vi "SubPanel_DataCollection_Rev11_v6.vi"(0 "DCPowerInformationClusterArray_Input":T6(array[cluster]), 1 "VISAPowerInfoInputArray":T5(array[cluster]), 2 "Run Data SubPanel Input":T4, 3 "RF Block Parameters":T3, 4 "Oscilloscope Info Array":T2(array[cluster]) {"vertical coupling" items=["AC", "DC", "Ground"]}, 6 "New Run?":bool, 7 "error in":errorcluster) -> (20 "DCPowerInformationClusterArray_Output":T6(array[cluster]), 21 "VISAPowerInfoInputOutput":T5(array[cluster]), 22 "Run Data SubPanel Output":T4, 23 "RF Block Parameters Output":T3, 24 "Oscilloscope Info Array Output":T2(array[cluster]) {"vertical coupling" items=["AC", "DC", "Ground"]}, 25 "Reinitialize?":bool, 26 "Data Was Collected?":bool, 27 "error out":errorcluster)   [LabVIEW 2019]
uses:
  Controls/DataBlockControl.ctl
  Controls/QueueDataControl_V3.ctl
  <vilib>/Utility/file.llb/Write Delimited Spreadsheet (string).vi
  Controls/RFBlockControl.ctl
  <instrlib>/niScope/Controls/niScope vertical coupling.ctl
panel:
  out "DCPowerInfoArray":string[][](array[string])
  out "Array":string[][][](array[string])
  out "Current Measurements":cluster{dbl[], dbl[]}[](graph)
  out "Voltage Measurements":cluster{dbl[], dbl[]}[](graph)
  out "Exiting":bool
  out "Full Run Information":string
  out "Ready For Next Run?":bool
  in  "Next Run":bool
  out "Recording Data":bool
  out "Current 2":waveform(dbl)[](graph)
  out "Voltage 2":waveform(dbl)[](graph)
  in  "Record Data Toggle":bool
  out "error of collection":errorcluster
  in  "force exit SubVI":bool
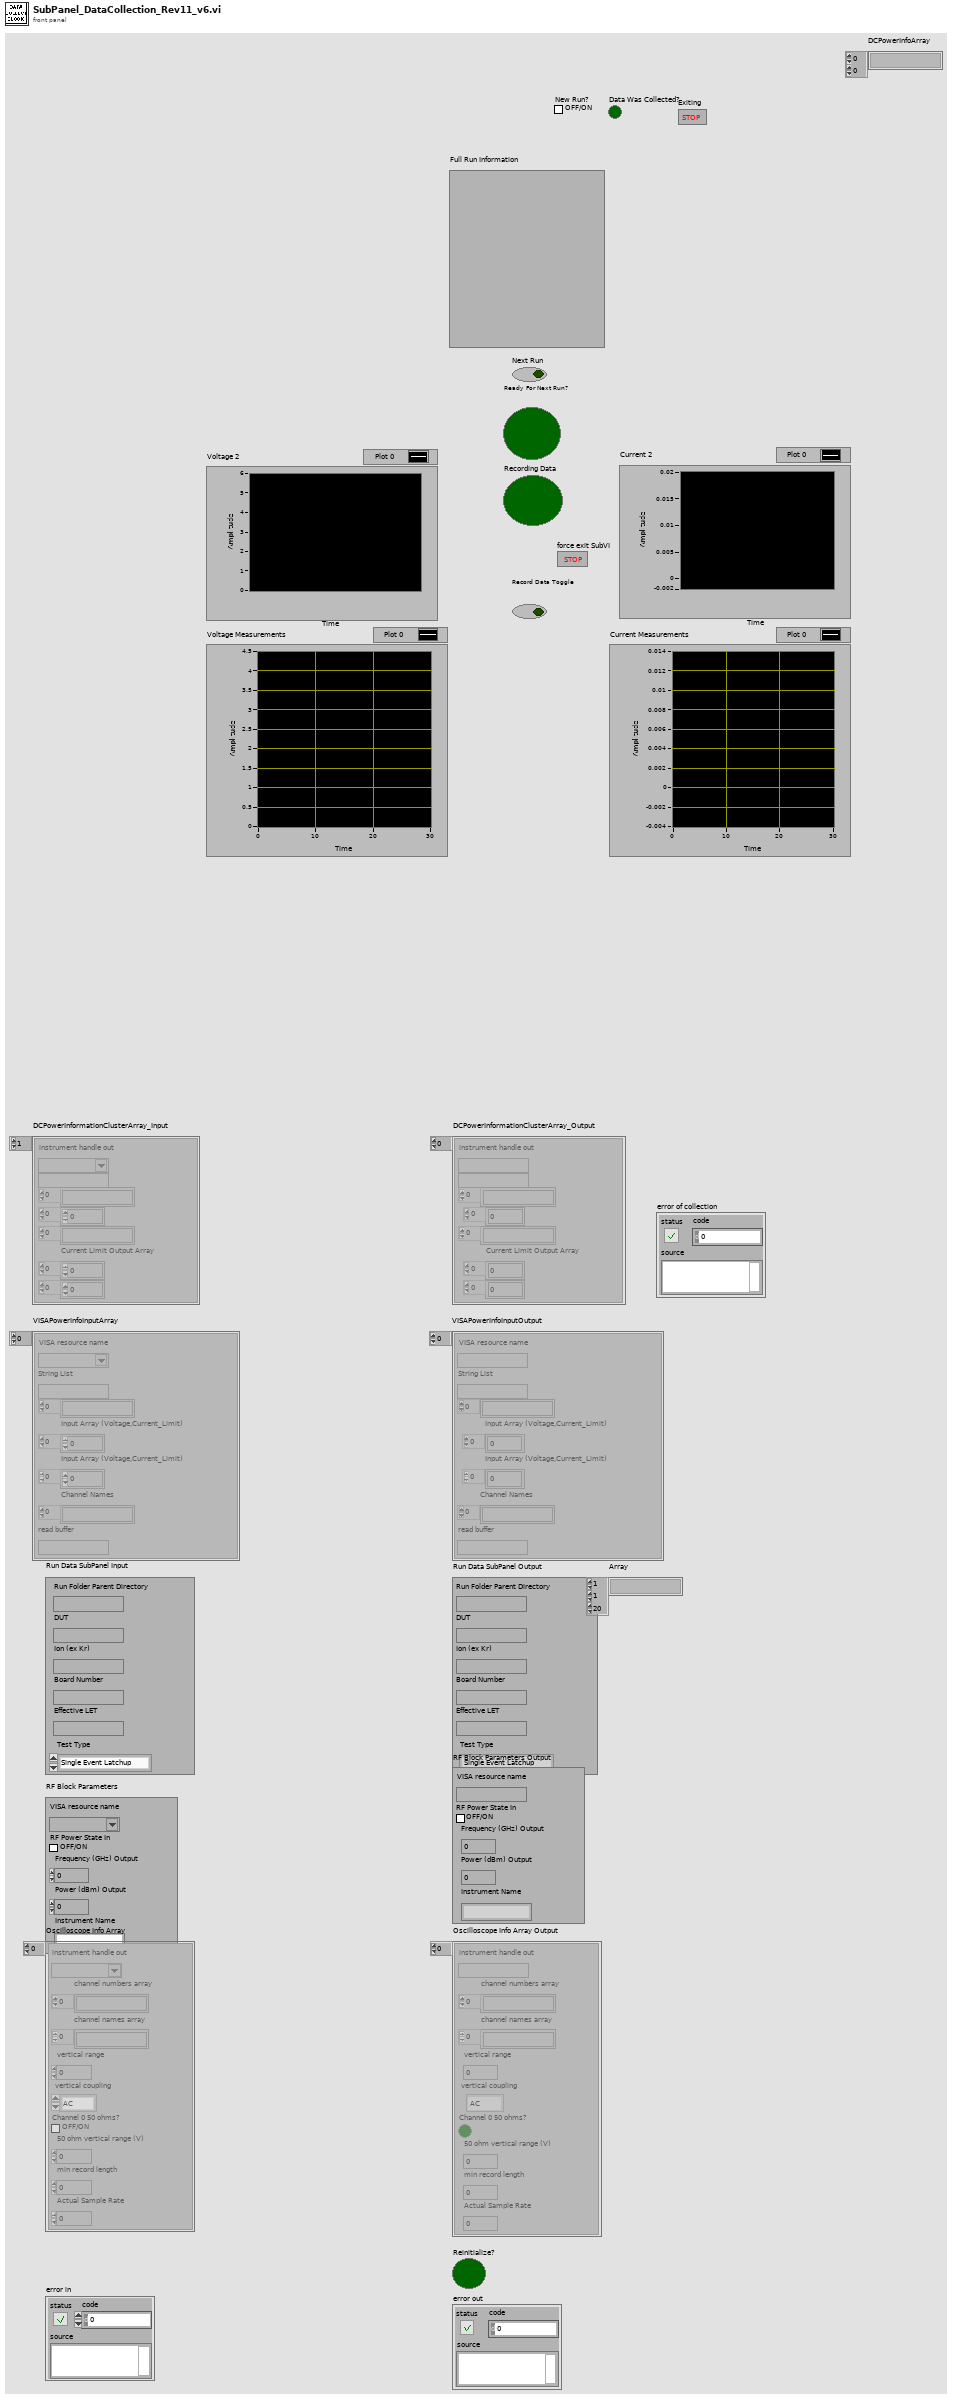
[diagram p1: front panel]
types:
  T1 = typedef "niScope vertical coupling.ctl" = i32
  T2 = cluster{"instrument handle out":refnum<k15>, "channel numbers array":string[], "channel names array":string[], "vertical range":dbl, "vertical coupling":T1, "Channel 0 50 ohms?":bool, "50 ohm vertical range (V)":dbl, "min record length":i32, "Actual Sample Rate":dbl}[]
  T3 = typedef "RFBlockControl.ctl" = cluster{"VISA resource name":refnum<visa-resource-name>, "RF Power State In":bool, "Frequency (GHz) Output":dbl, "Power (dBm) Output":dbl, "Instrument Name":string}
  T4 = typedef "DataBlockControl.ctl" = cluster{"Run Folder Parent Directory":path, "DUT":string, "Ion (ex Kr)":string, "Board Number":string, "Effective LET":string, "Test Type":enum16{"Single Event Latchup", "Single Event Transient", "Single Event Upset"}}
  T5 = cluster{"VISA resource name":refnum<visa-resource-name>, "String List":string, string[], "Input Array (Voltage,Current_Limit)":dbl[], "Input Array (Voltage,Current_Limit)":dbl[], "Channel Names":string[], "read buffer":string}[]
  T6 = cluster{"instrument handle out":refnum<k15>, string, string[], dbl[], string[], "Current Limit Output Array":dbl[], dbl[]}[]
  T7 = typedef "QueueDataControl_V3.ctl" = cluster{"Array of fetched data":dbl[][][], "Channel Names Array":string[], "Voltage Waveform Array":waveform(dbl)[], "Current Waveform Array":waveform(dbl)[], "Resetting Time":timestamp, "Beam Logic":dbl}
  T8 = cluster{"IVI Refnum out":refnum<k15>, string, "voltage level channel 23":dbl, "Channel Name 23":string, "Current Limit":dbl, "Measure Record dt":dbl, string}[]
  T9 = cluster{"created path":path, "DCPowerInformation_byChannel":cluster{"IVI Refnum out":refnum<k15>, string, "voltage level channel 23":dbl, "Channel Name 23":string, "Current Limit":dbl, "Measure Record dt":dbl, string}[], string[]}
  T10 = cluster{"Array of fetched data":dbl[][], string, i32[]}
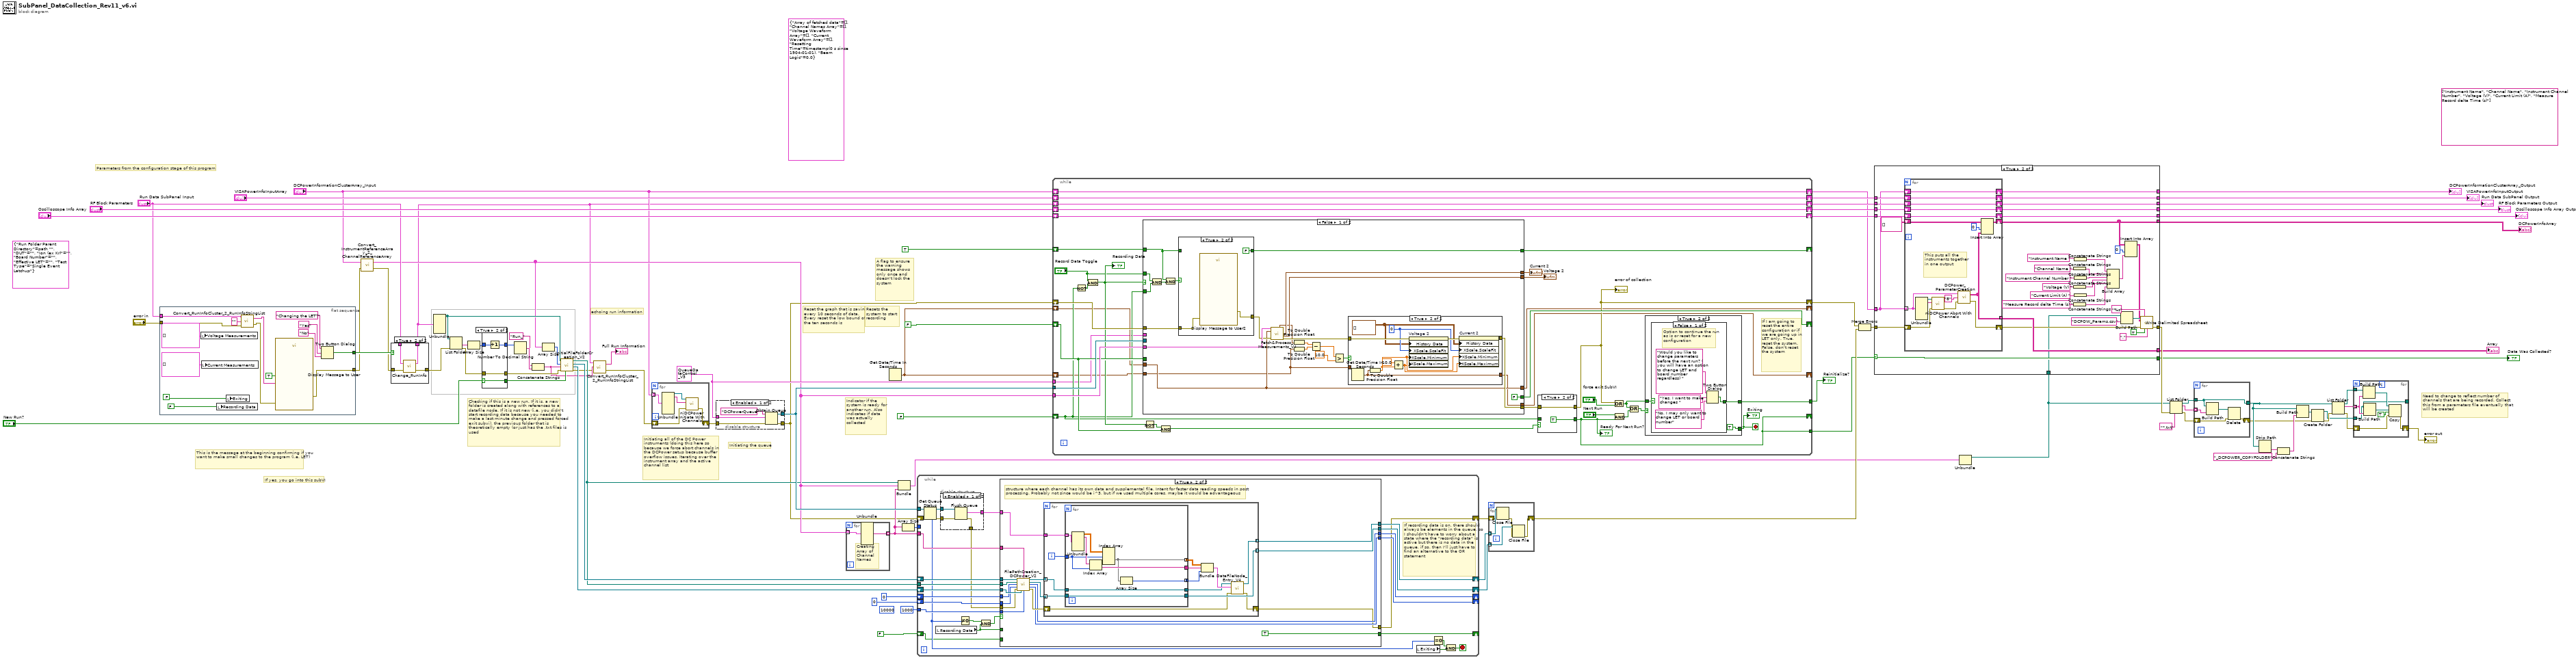
[diagram p0: block diagram]
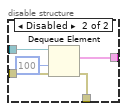
[diagram p2: hidden frame]
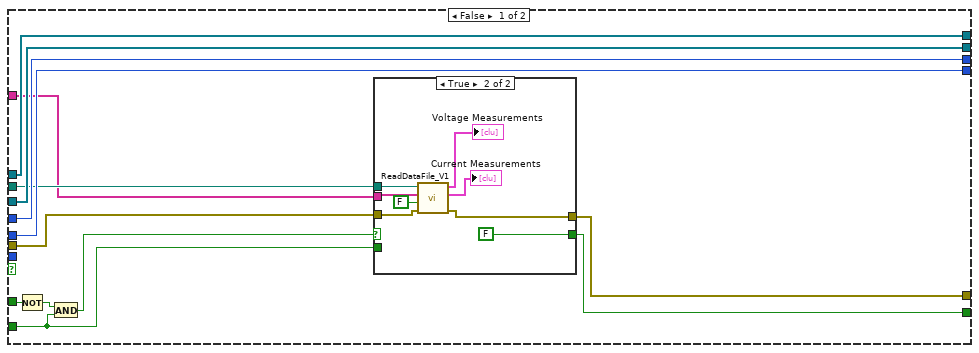
[diagram p3: hidden frame]
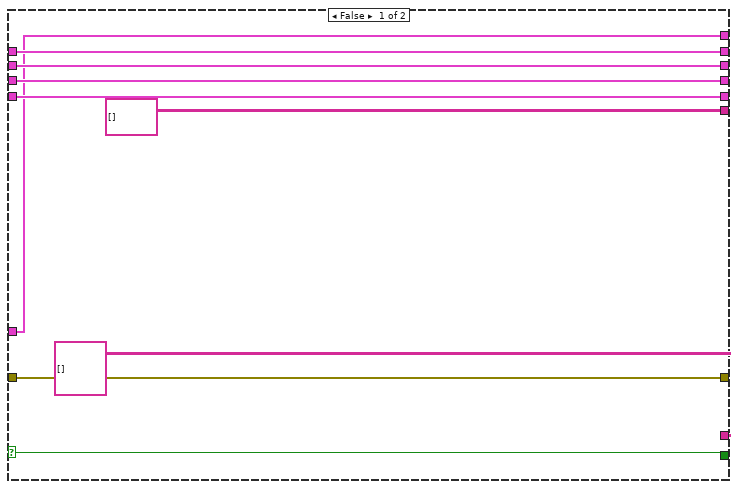
[diagram p5: hidden frame]
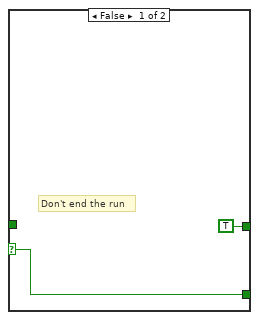
[diagram p9: hidden frame]
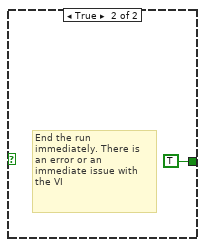
[diagram p10: hidden frame]
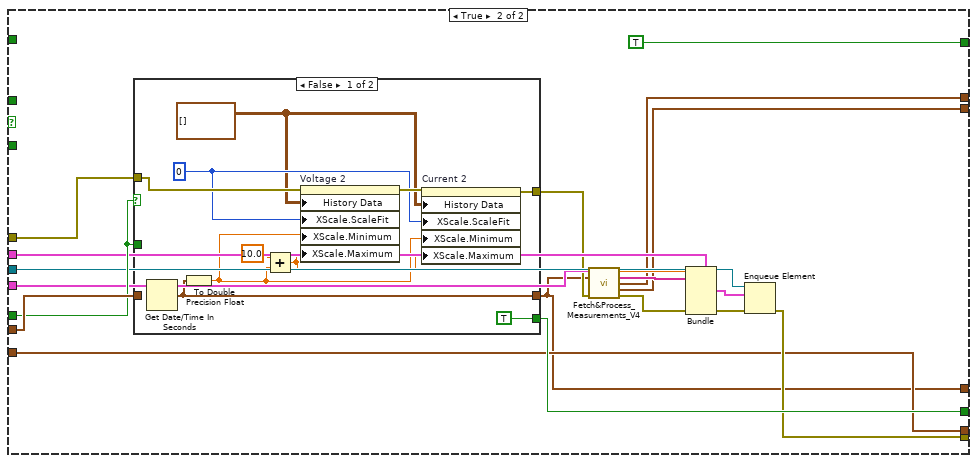
[diagram p14: hidden frame]
diagram:
  (unwired) string[] ["Instrument Name", "Channel Name", "Instrument Channel Number", "Voltage (V)", "Current Limit (A)", "Measure Record delta Time (s)"] ("new element/subarray")
  w54 = T7 {"Array of fetched data"=[], "Channel Names Array"=[], "Voltage Waveform Array"=[], "Current Waveform Array"=[], "Resetting Time"=timestamp(0 s since 1904-01-01), "Beam Logic"=0.0} ("DCPower Queue Data Double Array Format")
  (unwired) T7 {"Array of fetched data"=[], "Channel Names Array"=[], "Voltage Waveform Array"=[], "Current Waveform Array"=[], "Resetting Time"=timestamp(0 s since 1904-01-01), "Beam Logic"=0.0} ("DCPower Double Array Queue")
  (unwired) 10000 ("binary file indexor in")
  (unwired) T4 {"Run Folder Parent Directory"=path "", "DUT"="", "Ion (ex Kr)"="", "Board Number"="", "Effective LET"="", "Test Type"=enum."Single Event Latchup"} ("Run Data Configuration")
  # "Initiating the queue"
  # "echoing run information"
  # "Checking if this is a new run. If it is, a new folder is created along with references to a datafile node. If it is not new (i.e. you didn't start recording data because you needed to make a last minute change and pressed forced exit subvi), the previous folder that is theoretically empty (or just has the .txt files is used"
  # "If yes, you go into this subVI"
  # "This is the message at the beginning confirming if you want to make small changes to the program (i.e. LET)"
  # "Parameters from the configuration stage of this program"
  # "Reset the graph that is saving every 10 seconds of data. Every reset the low bound of the ten seconds is"
  # "Need to change to reflect number of channels that are being recorded. Collect this from a parameters file eventually that will be created"
  # "Indicator if the system is ready for another run. Also indicates if data was actually collected"
  # "Resets the system to start recording"
  # "A flag to ensure the warning message shows only once and doesn't lock the system"
  # "Initiating all of the DC Power instruments (doing this here so because we force abort channels in the DCPower setup because buffer overflow issues. Iterating over the instrument array and the active channel list"
  n1 = flat-sequence {
    tunnel: [w95] -> w70
    tunnel: "error in" -> [w87]
    tunnel: [w99] -> w75
    tunnel: "Run Data SubPanel Input" -> [w86]
    frame #0 {
      n2 = local write "Voltage Measurements"(cluster{dbl[], dbl[]}[] [] ("Voltage Measurements")) -> ()
      n3 = local write "Current Measurements"(cluster{dbl[], dbl[]}[] [] ("Current Measurements")) -> ()
      n4 = local write "Recording Data"(FALSE ("Recording Data")) -> ()
      n5 = local write "Exiting"(FALSE ("Forced Exit")) -> ()
      n6 = call "Convert_RunInfoCluster_2_RunInfoStringList.vi"("error in"=w87, "Run Number"="", "Run Data SubPanel Input"=w86) -> ("error output"=w88:errorcluster, "Run Data Output"=w89:string)
      n7 = call "Display Message to User"("error in (no error)"=w88, "Enable"=TRUE, "Message"=w89) -> ("error out"=w95:errorcluster)  [unwired: 7 in, 1 out]
      n8 = Two Button Dialog(message="Changing the LET?", 1:"No" ("F button name (\"Cancel\")"), 2:"Yes" ("T button name (\"OK\")")) -> (T button?=w99:bool)
    }
  }
  n9 = call "Convert_InstrumentReferenceArray_2_ChannelReferenceArray.vi"("error in (no error)"=w70, "DCPowerInformationClusterArray_Input"="DCPowerInformationClusterArray_Input") -> ("error out"=w69:errorcluster, "DCPowerInformation_byChannel"=w27:T8)
  n10 = case shown="True" w75 {
    tunnel: "Run Data SubPanel Input" -> [w101 w105]
    tunnel: [w101 w104] -> w4
    tunnel: [w100 w103] -> w71
    tunnel: w69 -> [w100 w102]
    frame False {
    }
    frame True {
      n11 = call "Change_RunInfo.vi"("error in (no error)"=w102, "Run Data SubPanel in"=w105) -> ("error out"=w103:errorcluster, "Run Data SubPanel out"=w104:T4)
    }
  }
  n12 = Unbundle(w4) -> ("Run Folder Parent Directory"=w72:path)  [unwired: 5 out]
  n13 = List Folder(path=w72, error in=w71) -> (folder names=w73:string[], error out=w57:errorcluster)  [unwired: 2 in, 2 out]
  n14 = Array Size(array=w73) -> (size(s)=w60:i32)
  n15 = case shown="True" "New Run?" {
    selector: "New Run?" -> [w107 w110]
    tunnel: [w108 w112] -> w61
    tunnel: w60 -> [w108 w111]
    tunnel: [w107 w110] -> w59
    tunnel: [w106 w109] -> w58
    tunnel: w57 -> [w106 w109]
    frame False {
    }
    frame True {
      n16 = Increment(x=w111) -> (x+1=w112:i32)
    }
  }
  n17 = Number To Decimal String(number=w61) -> (decimal integer string=w64:string)  [unwired: 1 in]
  n18 = Concatenate Strings("Run_", w64) -> (w3:string)
  n19 = Array Size(array=w27) -> (size(s)=w56:i32)
  n20 = call "InitialFileFolderCreation_V2.vi"("New Run?"=w59, "error in (no error)"=w58, "Run Number"=w3, "DCPowerArrayClusterSize"=w56, "base path"=w72) -> ("error out"=w2:errorcluster, "SupplementalDataFileReferenceObjectArray"=w67:refnum<file>[], "DataFileReferenceObjectArray"=w68:refnum<file>[], "created path"=w11:path)  [unwired: 3 in]
  n21 = call "Convert_RunInfoCluster_2_RunInfoStringList.vi"("error in"=w2, "Run Number"=w3, "Run Data SubPanel Input"=w4) -> ("error output"=w1:errorcluster, "Run Data Output"=→"Full Run Information":string)
  n22 = for {
    shift-right: [w113] -> w9
    shift-left: w1 -> [w115]
    tunnel: "DCPowerInformationClusterArray_Input" -> [w117] mode=indexing
    n23 = Unbundle(w117) -> ("instrument handle out"=w114:refnum<k15>, w116:string)  [unwired: 5 out]
    n24 = call <instrlib>:"niDCPower Initiate With Channels.vi"("error in (no error)"=w115, "channel name"=w116, "instrument handle"=w114) -> ("error out"=w113:errorcluster)  [unwired: 7 in, 1 out]
  }
  n25 = disable-structure shown="Enabled" {
    disable-tunnel: w9 -> [w121 w123]
    disable-tunnel: [w120 w123] -> w6
    disable-tunnel: [w119 _] -> w80
    disable-tunnel: w54 -> [w118 _]
    frame Enabled {
      n26 = Obtain Queue(name (unnamed)="DCPowerQueue", element data type=w118, error in (no error)=w121) -> (queue out=w119:refnum<queue>, error out=w120:errorcluster)  [unwired: 2 in, 1 out]
    }
    frame Disabled {
    }
  }
  n27 = for {
    tunnel: w27 -> [w125] mode=indexing
    tunnel: [w124] -> w28 mode=indexing
    # "Creating Array of Channel Names"
    n28 = Unbundle(w125) -> ("Channel Name 23"=w124:string)  [unwired: 6 out]
  }
  n29 = Get Date/Time In Seconds() -> (seconds since 1Jan1904=w7:timestamp)
  n30 = Bundle("created path"=w11, "DCPowerInformation_byChannel"=w27, w28) -> (w26:T9)  [unwired: 1 in]
  n31 = Array Size(array=w28) -> (size(s)=w49:i32)
  n32 = while {
    tunnel: w80 -> [w152]
    shift-right: [w139] -> w51
    shift-left: w6 -> [w151]
    tunnel: w11 -> [w148]
    shift-right: [w141] -> w53
    shift-left: w68 -> [w149]
    shift-right: [w140] -> w52
    shift-left: w67 -> [w147]
    shift-right: [w143] -> _
    shift-left: 0 ("binary file indexor in") -> [w146]
    shift-right: [w142] -> _
    shift-left: 0 ("binary file indexor in") -> [w145]
    tunnel: 1000 ("binary file indexor in") -> [w144]
    tunnel: w28 -> [w150]
    tunnel: w49 -> [_]
    shift-right: [w128] -> _
    shift-left: FALSE -> [w127]
    stop <- w136 stop-if-true
    # "If recording data is on, there should always be elements in the queue, so I shouldn't have to worry about a state where the \"recording data\" is active but there is no data in the queue, if so, then I'll just have to find an alternative to the OR statement"
    n33 = Get Queue Status(queue=w152, error in (no error)=w151) -> (queue out=w133:refnum<queue>, error out=w134:errorcluster, # elements in queue=w129:i32)  [unwired: 1 in, 5 out]
    n34 = local read "Recording Data"() -> (w126:bool)
    n35 = disable-structure shown="Enabled" {
      disable-tunnel: [w156 w158] -> w135
      disable-tunnel: w134 -> [w155 w160]
      disable-tunnel: w133 -> [w154 w161]
      disable-tunnel: [w153 w157] -> w132
      frame Enabled {
        n36 = Flush Queue(queue=w154, error in (no error)=w155) -> (remaining elements=w153:T7[], error out=w156:errorcluster)  [unwired: 1 out]
      }
      frame Disabled {
        n37 = Dequeue Element(queue=w161, timeout in ms (-1)=100, error in (no error)=w160) -> (element=w157:T7, error out=w158:errorcluster)  [unwired: 2 out]
      }
    }
    n38 = Not Equal To 0?(x=w129) -> (x != 0?=w131:bool)
    n39 = And(x=w131, y=w126) -> (x .and. y?=w130:bool)
    n40 = case shown="True" w130 {
      tunnel: w132 -> [_ w202]
      tunnel: w135 -> [w165 w196]
      tunnel: w150 -> [w166 w188]
      tunnel: w149 -> [w173 w201]
      tunnel: w148 -> [w167 w200]
      tunnel: w147 -> [w174 w199]
      tunnel: w146 -> [w172 w198]
      tunnel: w145 -> [w171 w187]
      tunnel: w144 -> [_ w186]
      tunnel: [w172 w195] -> w143
      tunnel: [w171 w194] -> w142
      tunnel: [w173 w191] -> w141
      tunnel: [w174 w190] -> w140
      tunnel: [w164 w189] -> w139
      tunnel: [w163 TRUE] -> w128
      tunnel: w127 -> [w162 _]
      tunnel: w126 -> [w170 _]
      frame False {
        n41 = Not(x=w170) -> (.not. x?=w169:bool)
        n42 = And(x=w169, y=w162) -> (x .and. y?=w168:bool)
        n43 = case shown="True" w168 {
          tunnel: w167 -> [_ w184]
          tunnel: w166 -> [_ w183]
          tunnel: w165 -> [w176 w181]
          tunnel: [w176 w180] -> w164
          tunnel: [w175 FALSE] -> w163
          tunnel: w162 -> [w175 _]
          frame False {
          }
          frame True {
            n44 = call "ReadDataFile_V1.vi"("error in (no error)"=w181, "Create CSV files?"=FALSE, "Channel Names Array"=w183, "DataFolder Path"=w184) -> ("error out"=w180:errorcluster, "Current Measurements"=→"Current Measurements":cluster{dbl[], dbl[]}[], "Voltage Measurements"=→"Voltage Measurements":cluster{dbl[], dbl[]}[])  [unwired: 5 in]
          }
        }
      }
      frame True {
        # "structure where each channel has its own data and supplemental file. Intent for faster data reading speeds in post processing. Probably not since would be i^3, but if we used multiple cores, maybe it would be advantageous"
        n45 = call "FilePathCreation_DCPower_V2.vi"("binary file input reference array 1"=w201, "Channel Name Input array"=w188, "data output directory folder"=w200, "binary file indexor in"=w198, "Reset counter in"=w187, "error in (no error)"=w196, "binary file input reference array 2"=w199, "reset threshold"=w186) -> ("binary file output reference array"=w193:refnum<file>[], "binary file output reference array 2"=w192:refnum<file>[], "binary file indexor out"=w195:i32, "reset counter out"=w194:i32, "error out"=w197:errorcluster)  [unwired: 3 in]
        n46 = for {
          shift-right: [w205] -> w189
          shift-left: w197 -> [w206]
          tunnel: w202 -> [w215]
          tunnel: w192 -> [w212] mode=indexing
          tunnel: w193 -> [w211] mode=indexing
          tunnel: [w210] -> w190 mode=indexing
          tunnel: [w204] -> w191 mode=indexing
          i -> [w209]
          n47 = for {
            tunnel: w215 -> [w224] mode=indexing
            tunnel: w209 -> [w221]
            tunnel: [w216] -> w203 mode=concatenating
            tunnel: [w220] -> w214
            tunnel: w212 -> [w219]
            tunnel: w211 -> [w217]
            tunnel: [w217] -> w207
            tunnel: [w219] -> w210
            tunnel: [w218] -> w213 mode=concatenating
            n48 = Unbundle(w224) -> ("Array of fetched data"=w223:dbl[][][], "Channel Names Array"=w222:string[])  [unwired: 4 out]
            n49 = Index Array(array=w222, index=w221) -> (element=w220:string)
            n50 = Index Array(array=w223, index (dim 0)=w221) -> (element=w216:dbl[][])  [unwired: 2 in]
            n51 = Array Size(array=w216) -> (size(s)=w218:i32[])
          }
          n52 = Bundle("Array of fetched data"=w203, w214, w213) -> (w208:T10)  [unwired: 1 in]
          n53 = call "DataFileNode_Entry_V4.vi"("error in (no error)"=w206, "Queued Elements"=w208, "Byte Stream File in"=w207) -> ("error out"=w205:errorcluster, "Byte Stream File out"=w204:refnum<file>)  [unwired: 7 in]
        }
      }
    }
    n54 = local read "Exiting"() -> (w138:bool)
    n55 = Equal To 0?(x=w129) -> (x = 0?=w137:bool)
    n56 = And(x=w137, y=w138) -> (x .and. y?=w136:bool)
  }
  n57 = while {
    shift-right: [w255] -> w16
    shift-left: "DCPowerInformationClusterArray_Input" -> [w255]
    shift-right: [w259] -> w18
    shift-left: "VISAPowerInfoInputArray" -> [w259]
    shift-right: [w258] -> w20
    shift-left: w4 -> [w258]
    shift-right: [w257] -> w22
    shift-left: "RF Block Parameters" -> [w257]
    shift-right: [w256] -> w24
    shift-left: "Oscilloscope Info Array" -> [w256]
    shift-right: [w240] -> w55
    shift-left: w6 -> [w253]
    tunnel: w27 -> [w254]
    shift-right: [w250] -> _
    shift-left: FALSE -> [w247]
    tunnel: w80 -> [w249]
    shift-right: [w229] -> _
    shift-left: FALSE -> [w234]
    tunnel: [w238] -> w79
    shift-right: [w232] -> _
    shift-left: TRUE ("x .and. y?") -> [w233]
    shift-right: [w230] -> _
    shift-left: w7 -> [w231]
    tunnel: [w229] -> w15
    tunnel: w54 -> [w227]
    shift-right: [w225] -> _
    shift-left: w7 -> [w226]
    stop <- w228 stop-if-true
    # "If I am going to reset the entire configuration or if we are going up in LET only. True, reset the system. False, don't reset the system"
    n58 = Not(x=w234) -> (.not. x?=w236:bool)
    n59 = And(x="Record Data Toggle", y=w236) -> (x .and. y?=w237:bool)
    "Recording Data" <- w237
    n60 = case shown="False" w237 {
      tunnel: w254 -> [w296 w320]
      tunnel: w253 -> [w293 w328]
      tunnel: [w282 w315] -> w252
      tunnel: [w283 w314] -> w251
      tunnel: w247 -> [_ w326]
      tunnel: [FALSE w327] -> w250
      tunnel: w249 -> [_ w325]
      tunnel: [w294 w324] -> w245
      tunnel: "Record Data Toggle" -> [w290 _]
      tunnel: w234 -> [w291 _]
      tunnel: w233 -> [w286 _]
      tunnel: [w287 TRUE] -> w232
      tunnel: w231 -> [w285 w329]
      tunnel: [w285 w318] -> w230
      tunnel: w227 -> [_ w323]
      tunnel: w226 -> [w281 w321]
      tunnel: [w284 w321] -> w225
      frame False {
        n61 = And(x=w290, y=w291) -> (x .and. y?=w289:bool)
        n62 = And(x=w286, y=w289) -> (x .and. y?=w288:bool)
        n63 = case shown="True" w288 {
          tunnel: [w309 w311] -> w292
          tunnel: w293 -> [w309 w312]
          tunnel: [w308 FALSE] -> w287
          tunnel: w286 -> [w308 _]
          frame False {
          }
          frame True {
            n64 = call "Display Message to User2"("error in (no error)"=w312) -> ("error out"=w311:errorcluster)  [unwired: 9 in, 1 out]
          }
        }
        n65 = call "Fetch&Process_Measurements_V4.vi"("DCPowerInformation_byChannel"=w296, "Initial Time"=w285, "error in (no error)"=w292) -> ("Latest Time"=w279:timestamp, "Current Waveform Array"=w282:waveform(dbl)[], "Voltage Waveform Array"=w283:waveform(dbl)[], "error out"=w280:errorcluster)  [unwired: 6 in, 3 out]
        n66 = To Double Precision Float(number=w279) -> (double precision float=w277:dbl)
        n67 = To Double Precision Float(number=w281) -> (double precision float=w278:dbl)
        n68 = Subtract(x=w277, y=w278) -> (x-y=w276:dbl)
        n69 = Greater?(x=w276, y=10.0) -> (0:w274:bool)
        n70 = case shown="True" w274 {
          tunnel: w280 -> [w297 w307]
          tunnel: [w298 w304] -> w284
          tunnel: w281 -> [w298 _]
          tunnel: [w297 w305] -> w294
          frame False {
          }
          frame True {
            w303 = u8 0 ("X Scale.Scale Fit")
            w302 = waveform(dbl)[][] [] ("History Data")
            n71 = Get Date/Time In Seconds() -> (seconds since 1Jan1904=w304:timestamp)
            n72 = To Double Precision Float(number=w304) -> (double precision float=w300:dbl)
            n73 = Add(x=10.0, y=w300) -> (x+y=w299:dbl)
            n74 = property on="Voltage 2" class="WFChart (strict)"(error in=w307, "History Data"=w302, "XScale.ScaleFit"=w303, "XScale.Minimum"=w300, "XScale.Maximum"=w299) -> (error out=w306:errorcluster)  [unwired: 1 in, 1 out]
            n75 = property on="Current 2" class="WFChart (strict)"(error in=w306, "History Data"=w302, "XScale.ScaleFit"=w303, "XScale.Minimum"=w300, "XScale.Maximum"=w299) -> (error out=w305:errorcluster)  [unwired: 1 in, 1 out]
          }
        }
      }
      frame True {
        n76 = case shown="False" w326 {
          tunnel: [w335 w343] -> w318
          tunnel: w329 -> [_ w343]
          tunnel: w328 -> [w340 w342]
          tunnel: [w338 w342] -> w319
          tunnel: [TRUE w341] -> w327
          tunnel: w326 -> [_ w341]
          frame False {
            w331 = waveform(dbl)[][] [] ("History Data")
            w336 = u8 0 ("X Scale.Scale Fit")
            n77 = Get Date/Time In Seconds() -> (seconds since 1Jan1904=w335:timestamp)
            n78 = To Double Precision Float(number=w335) -> (double precision float=w332:dbl)
            n79 = Add(x=10.0 ("y"), y=w332) -> (x+y=w334:dbl)
            n80 = property on="Voltage 2" class="WFChart (strict)"(error in=w340, "History Data"=w331, "XScale.ScaleFit"=w336, "XScale.Minimum"=w332, "XScale.Maximum"=w334) -> (error out=w339:errorcluster)  [unwired: 1 in, 1 out]
            n81 = property on="Current 2" class="WFChart (strict)"(error in=w339, "History Data"=w331, "XScale.ScaleFit"=w336, "XScale.Minimum"=w332, "XScale.Maximum"=w334) -> (error out=w338:errorcluster)  [unwired: 1 in, 1 out]
          }
          frame True {
          }
        }
        n82 = call "Fetch&Process_Measurements_V4.vi"("DCPowerInformation_byChannel"=w320, "Initial Time"=w318, "error in (no error)"=w319) -> ("Data As dbl Array"=w317:dbl[][][], "Channel Number Array"=w316:string[], "Current Waveform Array"=w315:waveform(dbl)[], "Voltage Waveform Array"=w314:waveform(dbl)[], "error out"=w313:errorcluster)  [unwired: 6 in, 2 out]
        n83 = Bundle(cluster=w323, "Array of fetched data"=w317, "Channel Names Array"=w316) -> (w322:T7)  [unwired: 4 in]
        n84 = Enqueue Element(queue=w325, element=w322, error in (no error)=w313) -> (error out=w324:errorcluster)  [unwired: 1 in, 2 out]
      }
    }
    "Voltage 2" <- w251
    "Current 2" <- w252
    n85 = Not(x=w237) -> (.not. x?=w248:bool)
    n86 = And(x=w248, y=w247) -> (x .and. y?=w246:bool)
    n87 = case shown="True" w246 {
      tunnel: w245 -> [w270 w272]
      tunnel: [w271 TRUE] -> w229
      tunnel: w234 -> [w271 _]
      tunnel: [w270 w272] -> w240
      frame False {
      }
      frame True {
      }
    }
    "error of collection" <- w240
    "Ready For Next Run?" <- w229
    n88 = Or(x=w240, y="force exit SubVI") -> (x .or. y?=w242:bool)
    n89 = And(x="Next Run", y=w229) -> (x .and. y?=w244:bool)
    n90 = Or(x=w242, y=w244) -> (x .or. y?=w243:bool)
    n91 = case shown="True" w243 {
      selector: w243 -> [w261 _]
      tunnel: w242 -> [_ w264]
      tunnel: [w261 TRUE] -> w228
      tunnel: [TRUE ("T button?") w262] -> w238
      frame False {
        # "Don't end the run"
      }
      frame True {
        n92 = case shown="False" w264 {
          tunnel: [w265 TRUE] -> w262
          frame False {
            # "Option to continue the run as is or reset for a new configuration"
            n93 = Two Button Dialog(message="Would you like to change parameters before the next run? ( you will have an option to change LET and board number regardless) ", 1:"No, I may only want to change LET or board number" ("F button name (\"Cancel\")"), 2:"Yes, I want to make changes " ("T button name (\"OK\")")) -> (T button?=w265:bool)
          }
          frame True {
            # "End the run immediately. There is an error or an immediate issue with the VI"
          }
        }
      }
    }
    "Exiting" <- w228
  }
  "Reinitialize?" <- w79
  n94 = for {
    tunnel: w53 -> [w348] mode=indexing
    tunnel: w52 -> [w346] mode=indexing
    shift-right: [w344] -> w50
    shift-left: w51 -> [w347]
    n95 = Close File(refnum=w348, error in=w347) -> (error out=w345:errorcluster)  [unwired: 1 out]
    n96 = Close File(refnum=w346, error in=w345) -> (error out=w344:errorcluster)  [unwired: 1 out]
  }
  n97 = Merge Errors(w55, w50) -> (w30:errorcluster)
  n98 = Unbundle(w26) -> ("created path"=w10:path)  [unwired: 2 out]
  n99 = case shown="True" w15 {
    selector: w15 -> [w352 w384]
    tunnel: w30 -> [w351 w395]
    tunnel: [w351 w378] -> w29
    tunnel: [w357 w394] -> w25
    tunnel: w24 -> [w357 w393]
    tunnel: [w356 w392] -> w23
    tunnel: w22 -> [w356 w391]
    tunnel: [w355 w390] -> w21
    tunnel: w20 -> [w355 w389]
    tunnel: [w354 w388] -> w19
    tunnel: w18 -> [w354 w387]
    tunnel: [w353 w386] -> w17
    tunnel: w16 -> [w353 w385]
    tunnel: [w352 w384] -> w14
    tunnel: [string[][][] [] w383] -> w13
    tunnel: [string[][] [] ("DCPowerInfoArray") w373] -> w12
    tunnel: w10 -> [_ w376]
    frame False {
    }
    frame True {
      n100 = for {
        shift-right: [w397] -> w379
        shift-left: w395 -> [w409]
        tunnel: w385 -> [w400] mode=indexing
        shift-right: [w408] -> w394
        shift-left: w393 -> [w408]
        shift-right: [w407] -> w392
        shift-left: w391 -> [w407]
        shift-right: [w406] -> w390
        shift-left: w389 -> [w406]
        shift-right: [w405] -> w388
        shift-left: w387 -> [w405]
        shift-right: [w404] -> w386
        shift-left: w385 -> [w404]
        tunnel: [w396] -> w383 mode=indexing
        shift-right: [w402] -> w373
        shift-left: string[][] [] ("DCPowerInfoArray") -> [w403]
        # "This puts all the instruments together in one output"
        n101 = Unbundle(w400) -> ("instrument handle out"=w411:refnum<k15>, w410:string)  [unwired: 5 out]
        n102 = call <instrlib>:"niDCPower Abort With Channels.vi"("error in (no error)"=w409, "channel name"=w410, "instrument handle"=w411) -> ("error out"=w398:errorcluster)  [unwired: 7 in, 1 out]
        n103 = call "DCPower_ParameterCreation.vi"("error in"=w398, "Precision"="8", "DCPowerInformationByInstrument"=w400) -> ("error out"=w397:errorcluster, "DCPowerInfoArray"=w396:string[][])
        n104 = Insert Into Array(array=w403, index (col)=0 ("disabled index (col)"), new element=w396) -> (w402:string[][])  [unwired: 1 in]
      }
      n105 = Concatenate Strings("Channel Name " ("string")) -> (w368:string)
      n106 = Concatenate Strings("Voltage (V) " ("string")) -> (w370:string)
      n107 = Concatenate Strings("Measure Record delta Time (s) " ("string")) -> (w372:string)
      n108 = Concatenate Strings("Instrument Name " ("string")) -> (w367:string)
      n109 = Concatenate Strings("Instrument Channel Number " ("string")) -> (w369:string)
      n110 = Concatenate Strings("Current Limit (A) " ("string")) -> (w371:string)
      n111 = Build Array(w367, w368, w369, w370, w371, w372) -> (w360:string[])
      n112 = Build Path(base path=w376, name or relative path="DCPOW_Params.csv") -> (appended path=w377:path)
      n113 = Insert Into Array(array=w373, index (col)=0 ("disabled index (col)"), new element=w360) -> (w359:string[][])  [unwired: 1 in]
      n114 = call-poly <vilib>:"Write Delimited Spreadsheet.vi"("file path (dialog if empty)"=w377, "format (%s)"="%s" ("format (%.3f)"), "2D data"=w359, "error in (no error)"=w379, "transpose? (no:F)"=TRUE, "delimiter (\\t)"="," ("delimiter (\\t)")) -> ("error out"=w378:errorcluster)  [unwired: 8 in, 1 out]
    }
  }
  "DCPowerInformationClusterArray_Output" <- w17
  "VISAPowerInfoInputOutput" <- w19
  "Run Data SubPanel Output" <- w21
  "RF Block Parameters Output" <- w23
  "Oscilloscope Info Array Output" <- w25
  "Data Was Collected?" <- w14
  "Array" <- w13
  "DCPowerInfoArray" <- w12
  n115 = List Folder(path=w10, pattern="*.txt", error in=w29) -> (path out=w35:path, filenames=w34:string[], error out=w33:errorcluster)  [unwired: 1 in, 1 out]
  n116 = for {
    tunnel: [w412] -> w36
    tunnel: w35 -> [w412]
    tunnel: w34 -> [w414] mode=indexing
    shift-right: [w415] -> w32
    shift-left: w33 -> [w416]
    n117 = Build Path(base path=w412, name or relative path=w414) -> (appended path=w413:path)
    n118 = Delete(path (use dialog)=w413, error in=w416) -> (error out=w415:errorcluster)  [unwired: 3 in, 2 out]
  }
  n119 = Strip Path(path=w36) -> (name=w40:string)  [unwired: 1 out]
  n120 = Concatenate Strings(w40, "_DCPOWER_COPYFOLDER" ("name or relative path")) -> (w38:string)
  n121 = Build Path(base path=w36, name or relative path=w38) -> (appended path=w47:path)
  n122 = Create Folder(path (use dialog)=w47, error in=w32) -> (created path=w42:path, error out=w45:errorcluster)  [unwired: 1 in, 1 out]
  n123 = List Folder(path=w36, error in=w45) -> (path out=w44:path, filenames=w43:string[], error out=w41:errorcluster)  [unwired: 2 in, 1 out]
  n124 = for {
    tunnel: w44 -> [w422]
    tunnel: w43 -> [w421] mode=indexing
    tunnel: w42 -> [w417]
    shift-right: [w424] -> w46
    shift-left: w41 -> [w418]
    tunnel: [w417] -> _
    n125 = Build Path(base path=w422, name or relative path=w421) -> (appended path=w419:path)
    n126 = Build Path(base path=w417, name or relative path=w421) -> (appended path=w420:path)
    n127 = Copy(8:w418, 9:TRUE ("overwrite (F)"), 10:w420, 11:w419) -> (0:w424:errorcluster)  [unwired: 1 in, 2 out]
  }
  "error out" <- w46
